vi "data_conversion.vi"(9 "input cluster":T2, 10 "Test mode":string, 11 "Delay time":string) -> (0 "Rsrc name for 19573":refnum<visa-resource-name>, 1 "Rsrc name for 19572":refnum<visa-resource-name>, 2 "Mode":T1(ring), 3 "Delay":dbl)   [LabVIEW 2015]
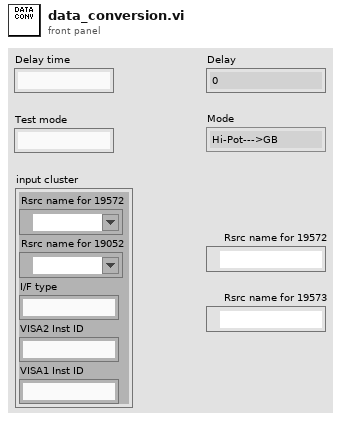
[diagram p1: front panel]
types:
  T1 = enum16{"Hi-Pot--->GB", "GB--->Hi-Pot", "Hi-Pot only", "GB only"}
  T2 = cluster{"Rsrc name for 19572":refnum<visa-resource-name>, "Rsrc name for 19052":refnum<visa-resource-name>, "I/F type":string, "VISA2 Inst ID":string, "VISA1 Inst ID":string}
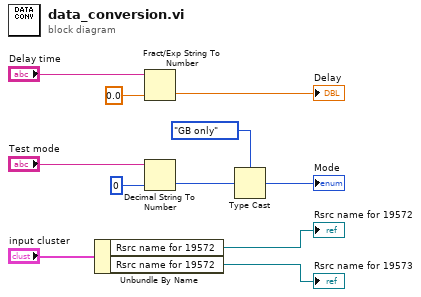
[diagram p0: block diagram]
diagram:
  n1 = Unbundle By Name("input cluster") -> ("Rsrc name for 19572"=→"Rsrc name for 19572":refnum<visa-resource-name>, "Rsrc name for 19572"=→"Rsrc name for 19573":refnum<visa-resource-name>)
  n2 = Fract/Exp String To Number(string="Delay time", default (0 dbl)=0.0 ("default (0 DBL)")) -> (number=→"Delay":dbl)  [unwired: 2 in, 1 out]
  n3 = Decimal String To Number(string="Test mode", default (0L)=i16 0 ("default (0 I32)")) -> (number=w9:i16)  [unwired: 1 in, 1 out]
  n4 = Type Cast(type=T1."GB only" ("Mode"), x=w9) -> (*(type *) &x=→"Mode":T1)
